vi "Find String Identifier.vi"(0 "input string":string) -> (1 "before string":string, 2 "remaining string":string, 3 "identifier":string)   [LabVIEW 2018, in "NI_Gmath.lvlib"]
uses:
  NI_Gmath.lvlib
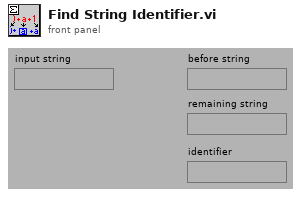
[diagram p1: front panel]
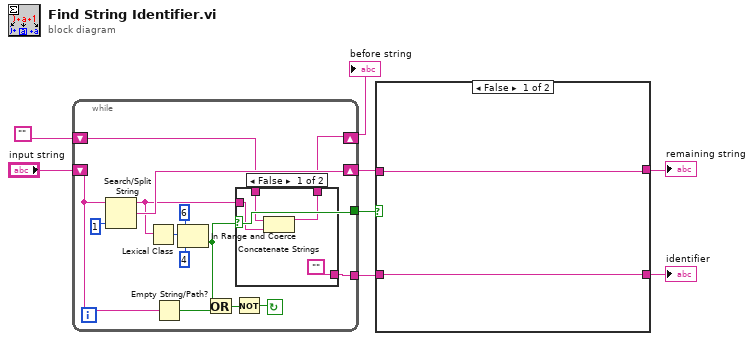
[diagram p0: block diagram]
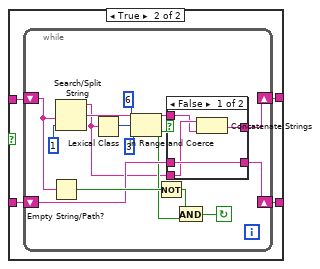
[diagram p3: hidden frame]
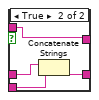
[diagram p4: hidden frame]
diagram:
  n1 = while {
    tunnel: [w12] -> w1
    shift-left: "" -> [w11]
    shift-right: [w10] -> w2
    shift-left: "input string" -> [w16]
    shift-right: [w18] -> w5
    tunnel: [w13] -> w3
    stop <- w17 continue-if-true
    n2 = Search/Split String(string=w16, offset (0)=1) -> (substring before match=w9:string, match + rest of string=w18:string)  [unwired: 1 in, 1 out]
    n3 = Lexical Class(1:w9) -> (0:w22:i16)
    n4 = Empty String/Path?(string/path=w16) -> (empty?=w15:bool)
    n5 = In Range and Coerce(upper limit=6 ("hi"), x=w22, lower limit=4 ("lo")) -> (In Range?=w13:bool)  [unwired: 1 out]
    n6 = Or(x=w13, y=w15) -> (x .or. y?=w14:bool)
    n7 = Not(x=w14) -> (.not. x?=w17:bool)
    n8 = case shown="False" w13 {
      tunnel: ["" w28] -> w12
      tunnel: w9 -> [w24 w28]
      tunnel: w11 -> [w25 w27]
      tunnel: [w23 w27] -> w10
      frame False {
        n9 = Concatenate Strings(w25, w24) -> (w23:string)
      }
      frame True {
      }
    }
  }
  "before string" <- w2
  n10 = case shown="False" w3 {
    tunnel: [w29 w34] -> w7
    tunnel: [w30 w33] -> w8
    tunnel: w5 -> [w29 w32]
    tunnel: w1 -> [w30 w31]
    frame False {
    }
    frame True {
      n11 = while {
        shift-left: w32 -> [w36]
        shift-right: [w43] -> w34
        shift-left: w31 -> [w42]
        shift-right: [w41] -> w33
        stop <- w37 continue-if-true
        n12 = Empty String/Path?(string/path=w36) -> (empty?=w45:bool)
        n13 = Search/Split String(string=w36, offset (0)=1) -> (substring before match=w35:string, match + rest of string=w40:string)  [unwired: 1 in, 1 out]
        n14 = Lexical Class(1:w35) -> (0:w48:i16)
        n15 = In Range and Coerce(upper limit=6 ("hi"), x=w48, lower limit=3 ("lo")) -> (In Range?=w38:bool)  [unwired: 1 out]
        n16 = Not(x=w45) -> (.not. x?=w39:bool)
        n17 = case shown="False" w38 {
          tunnel: [w51 w53] -> w43
          tunnel: w42 -> [w52 w55]
          tunnel: [w52 w54] -> w41
          tunnel: w35 -> [w50 w56]
          tunnel: w40 -> [w49 w53]
          frame False {
            n18 = Concatenate Strings(w50, w49) -> (w51:string)
          }
          frame True {
            n19 = Concatenate Strings(w55, w56) -> (w54:string)
          }
        }
        n20 = And(x=w39, y=w38) -> (x .and. y?=w37:bool)
      }
    }
  }
  "remaining string" <- w7
  "identifier" <- w8
